vi "Inform.vi"(8 "error in (no error)":errorcluster, 10 "Message in":refnum<class "InformMessage.lvclass">, 11 "Chat in":refnum<class "Chat.lvclass">) -> (0 "error out":errorcluster, 3 "Chat out":refnum<class "Chat.lvclass">)   [LabVIEW 2012, in "Chat.lvclass"]
doc: "The inform method processes the command inform'. \n\nThe command inform' is used for obtaining the latest instance data of the class. It also handles the current state of the observee and sets the 'ready' flag for the observee."
uses:
  Chat.lvclass
  <vilib>/Distrio/Murmex/InformMessage/InformMessage.lvclass
  <vilib>/Distrio/Murmex/Murmex/Murmex.lvclass
  <vilib>/Distrio/Murmex/Murmex/observer_cluster_2.ctl
  <vilib>/Distrio/Murmex/Murmex/observe_mode_enum.ctl
  <vilib>/Distrio/Murmex/Murmex/Queue type enum.ctl
  <vilib>/Distrio/Murmex/Murmex/Get component name.vi
  <vilib>/Distrio/Murmex/Murmex/Get ID.vi
  <vilib>/Distrio/Murmex/Murmex/Get observers.vi
  <vilib>/Distrio/Murmex/InformMessage/Get component name.vi
  <vilib>/Distrio/Murmex/Message/Get sender ID.vi
  <vilib>/Distrio/Murmex/Message/Get timestamp.vi
  <vilib>/Distrio/Murmex/Murmex/Set observers.vi
  <vilib>/Distrio/Murmex/Message/Message.lvclass
panel:
  # "This method is called when the INFORM\ntrigger is sent. \n\nOverride this method when your component needs to\nrespond to this trigger. \n\nCall parent for proper implementation"
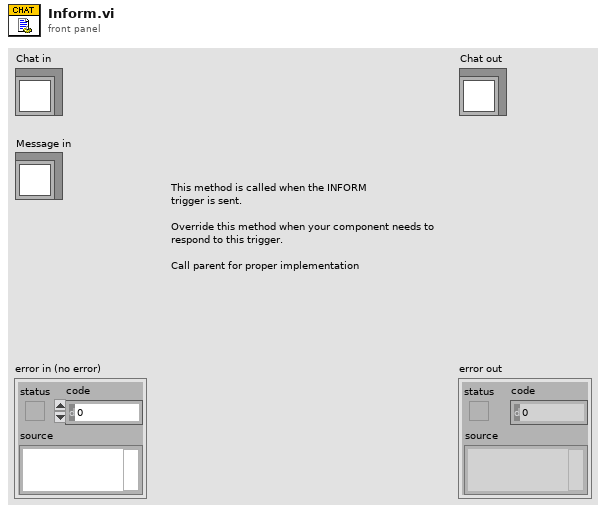
[diagram p1: front panel]
types:
  T1 = typedef "Murmex.lvlib/Murmex.lvclass/observer_cluster_2.ctl" = cluster{"ID":string, "observe mode":T2, "channels":string, "queue type":T3, "wait until done?":bool}
  T2 = typedef "Murmex.lvlib/Murmex.lvclass/observe_mode_enum.ctl" = enum16{"all data blocks", "only finished data blocks"}
  T3 = typedef "Murmex.lvlib/Murmex.lvclass/Queue type enum.ctl" = enum16{"RabbitMQ", "Network streaming queue"}
  T4 = typedef "Murmex.lvlib/Murmex.lvclass/command_enum.ctl" = enum16{"null", "initialise", "reset", "terminate", "acknowledge", "update", "inspect", "inform", "proceed", "start", "stop", "fetch", "configure", "generic"}
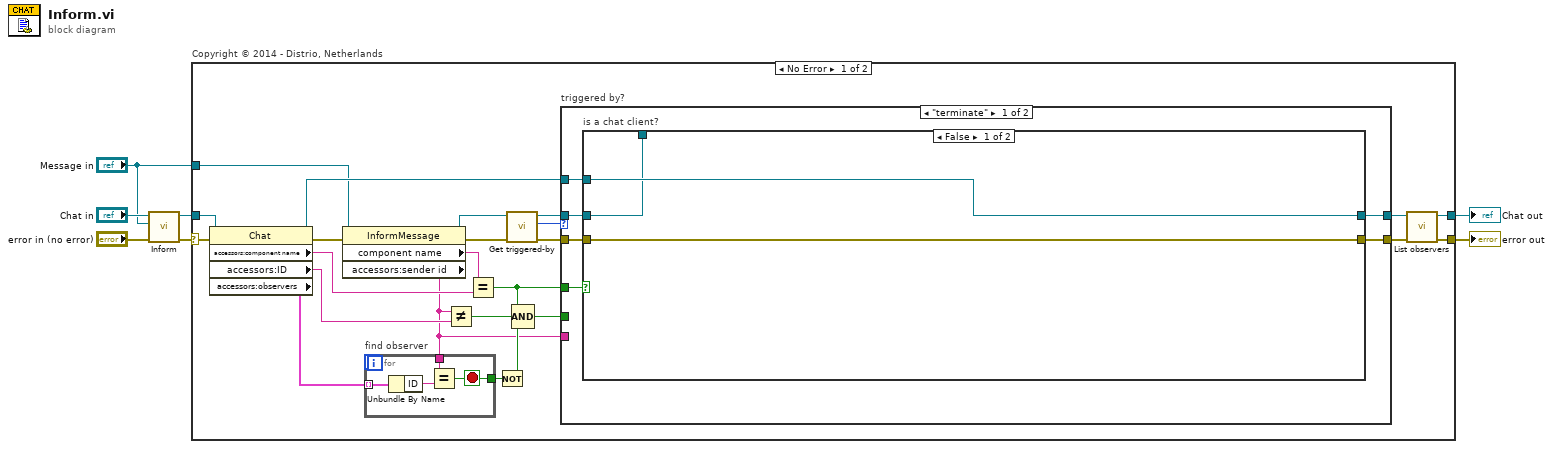
[diagram p0: block diagram]
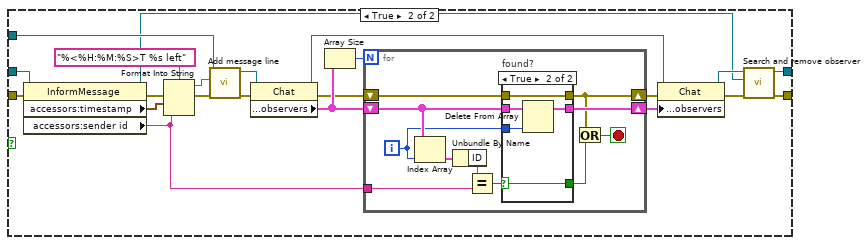
[diagram p2: hidden frame]
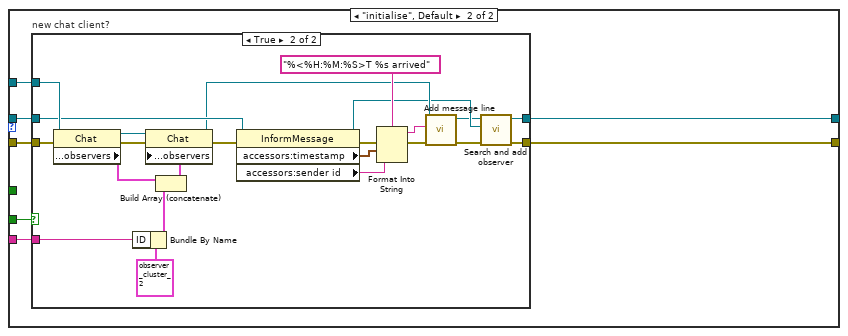
[diagram p4: hidden frame]
diagram:
  n1 = call-parent "Inform.vi"("error in (no error)"="error in (no error)", "Message in"="Message in", "Murmex in"="Chat in") -> ("error out"=w1:errorcluster, "Murmex out"=w4:refnum<class "Chat.lvclass">)  [unwired: 7 in]
  n2 = case "Copyright © 2014 - Distrio, Netherlands" shown="No Error" w1 {
    selector: w1 -> [w19 w119]
    tunnel: "Message in" -> [w20 _]
    tunnel: w4 -> [w31 w118]
    tunnel: [w11 w119] -> w3
    tunnel: [w9 w118] -> w2
    frame No Error {
      n3 = property class="Chat"(reference=w31, error in=w19) -> (reference out=w22:refnum<class "Chat.lvclass">, error out=w30:errorcluster, "accessors:component name"=w27:string, "accessors:ID"=w28:string, "accessors:observers"=w23:T1[])
      n4 = property class="InformMessage"(reference=w20, error in=w30) -> (reference out=w17:refnum<class "InformMessage.lvclass">, error out=w18:errorcluster, "component name"=w29:string, "accessors:sender id"=w21:string)
      n5 = for "find observer" {
        tunnel: w23 -> [w117] mode=indexing
        tunnel: w21 -> [w115]
        tunnel: [w114] -> w25
        stop <- w114 stop-if-true
        n6 = Unbundle By Name(w117) -> ("ID"=w116:string)
        n7 = Equal?(x=w115, y=w116) -> (x = y?=w114:bool)
      }
      n8 = Not Equal?(x=w21, y=w28) -> (x != y?=w13:bool)
      n9 = Equal?(x=w29, y=w27) -> (x = y?=w12:bool)
      n10 = Not(x=w25) -> (.not. x?=w24:bool)
      n11 = call <vilib>:"Get triggered-by.vi"("error in (no error)"=w18, "Message in"=w17) -> ("error out"=w15:errorcluster, "triggered-by"=w14:T4, "Message out"=w16:refnum<class "InformMessage.lvclass">)  [unwired: 7 in]
      n12 = Compound Arithmetic op=AND(w12, w13, w24) -> (w26:bool)
      n13 = case "triggered by?" shown="\"terminate\"" w14 {
        tunnel: [w34 w88] -> w10
        tunnel: [w33 w87] -> w8
        tunnel: w26 -> [_ w86]
        tunnel: w22 -> [w36 w85]
        tunnel: w21 -> [_ w84]
        tunnel: w16 -> [w35 w83]
        tunnel: w15 -> [w37 w82]
        tunnel: w12 -> [w32 _]
        frame "terminate" {
          n14 = case "is a chat client?" shown="False" w32 {
            tunnel: w37 -> [w39 w62]
            tunnel: w36 -> [w40 w48]
            tunnel: w35 -> [w38 w61]
            tunnel: [w39 w42] -> w34
            tunnel: [w40 w44] -> w33
            tunnel: [w38 _] -> _
            frame False {
            }
            frame True {
              n15 = property class="InformMessage"(reference=w61, error in=w62) -> (reference out=w41:refnum<class "InformMessage.lvclass">, error out=w58:errorcluster, "accessors:timestamp"=w60:timestamp, "accessors:sender id"=w55:string)
              n16 = Format Into String(format string="%<%H:%M:%S>T %s left", error in=w58, w60, w55) -> (resulting string=w49:string, error out=w50:errorcluster)  [unwired: 1 in]
              n17 = call "Add message line.vi"("error in (no error)"=w50, "Message in"=w49, "Chat in"=w48) -> ("error out"=w47:errorcluster, "Chat out"=w46:refnum<class "Chat.lvclass">)  [unwired: 7 in]
              n18 = property class="Chat"(reference=w46, error in=w47) -> (reference out=w53:refnum<class "Chat.lvclass">, error out=w51:errorcluster, "accessors:observers"=w57:T1[])
              n19 = Array Size(array=w57) -> (size(s)=w56:i32)
              n20 = for {
                N: w56 -> [_]
                shift-right: [w68] -> w54
                shift-left: w57 -> [w69]
                tunnel: w55 -> [w71]
                shift-right: [w65] -> w52
                shift-left: w51 -> [w66]
                i -> [w67]
                stop <- w63 stop-if-true
                n21 = Index Array(array=w69, index=w67) -> (element=w73:T1)
                n22 = Unbundle By Name(w73) -> ("ID"=w72:string)
                n23 = Equal?(x=w72, y=w71) -> (x = y?=w70:bool)
                n24 = case "found?" shown="True" w70 {
                  selector: w70 -> [w74 w77]
                  tunnel: w69 -> [w76 w81]
                  tunnel: [w76 w79] -> w68
                  tunnel: w67 -> [_ w80]
                  tunnel: [w75 w78] -> w65
                  tunnel: w66 -> [w75 w78]
                  tunnel: [w74 w77] -> w64
                  frame False {
                  }
                  frame True {
                    n25 = Delete From Array(array=w81, index=w80) -> (array with subset deleted=w79:T1[])  [unwired: 1 in, 1 out]
                  }
                }
                n26 = Or(x=w65, y=w64) -> (x .or. y?=w63:bool)
              }
              n27 = property class="Chat"(reference=w53, error in=w52, "accessors:observers"=w54) -> (reference out=w45:refnum<class "Chat.lvclass">, error out=w43:errorcluster)
              n28 = call "Search and remove observer.vi"("error in (no error)"=w43, "Message in"=w41, "Chat in"=w45) -> ("error out"=w42:errorcluster, "Chat out"=w44:refnum<class "Chat.lvclass">)  [unwired: 7 in]
            }
          }
        }
        frame "initialise", Default {
          n29 = case "new chat client?" shown="True" w86 {
            tunnel: w85 -> [w89 w108]
            tunnel: w82 -> [w90 w106]
            tunnel: [w90 w93] -> w88
            tunnel: [w89 w91] -> w87
            tunnel: w84 -> [_ w112]
            tunnel: w83 -> [_ w100]
            frame False {
            }
            frame True {
              n30 = property class="Chat"(reference=w108, error in=w106) -> (reference out=w107:refnum<class "Chat.lvclass">, error out=w105:errorcluster, "accessors:observers"=w109:T1[])
              n31 = Bundle By Name(cluster=T1 {"ID"="", "observe mode"=enum."all data blocks", "channels"="", "queue type"=enum."RabbitMQ", "wait until done?"=FALSE} ("observer"), "ID"=w112) -> (w111:T1)
              n32 = Build Array (concatenate)(w109, w111) -> (w110:T1[])
              n33 = property class="Chat"(reference=w107, error in=w105, "accessors:observers"=w110) -> (reference out=w97:refnum<class "Chat.lvclass">, error out=w99:errorcluster)
              n34 = property class="InformMessage"(reference=w100, error in=w99) -> (reference out=w95:refnum<class "InformMessage.lvclass">, error out=w101:errorcluster, "accessors:timestamp"=w104:timestamp, "accessors:sender id"=w103:string)
              n35 = Format Into String(format string="%<%H:%M:%S>T %s arrived", error in=w101, w104, w103) -> (resulting string=w96:string, error out=w98:errorcluster)  [unwired: 1 in]
              n36 = call "Add message line.vi"("error in (no error)"=w98, "Message in"=w96, "Chat in"=w97) -> ("error out"=w94:errorcluster, "Chat out"=w92:refnum<class "Chat.lvclass">)  [unwired: 7 in]
              n37 = call "Search and add observer.vi"("error in (no error)"=w94, "Message in"=w95, "Chat in"=w92) -> ("error out"=w93:errorcluster, "Chat out"=w91:refnum<class "Chat.lvclass">)  [unwired: 7 in]
            }
          }
        }
      }
      n38 = call "List observers.vi"("error in (no error)"=w10, "Chat in"=w8) -> ("error out"=w11:errorcluster, "Chat out"=w9:refnum<class "Chat.lvclass">)  [unwired: 8 in]
    }
    frame Error {
    }
  }
  "error out" <- w3
  "Chat out" <- w2
